vi "DELETE_clear_error_bulk.vi"(8 "API Key":string="cheia04042025tema2restfulapi", 11 "url":string="http://localhost:5000/ecu?param=clear_error_memory") -> (0 "delete_error_":string, 1 "DELETE_clear_specific_error_header":string)   [LabVIEW 2024]
uses:
  <vilib>/httpClient/LabVIEWHTTPClient.lvlib
panel:
  out "error out delete error memory":errorcluster
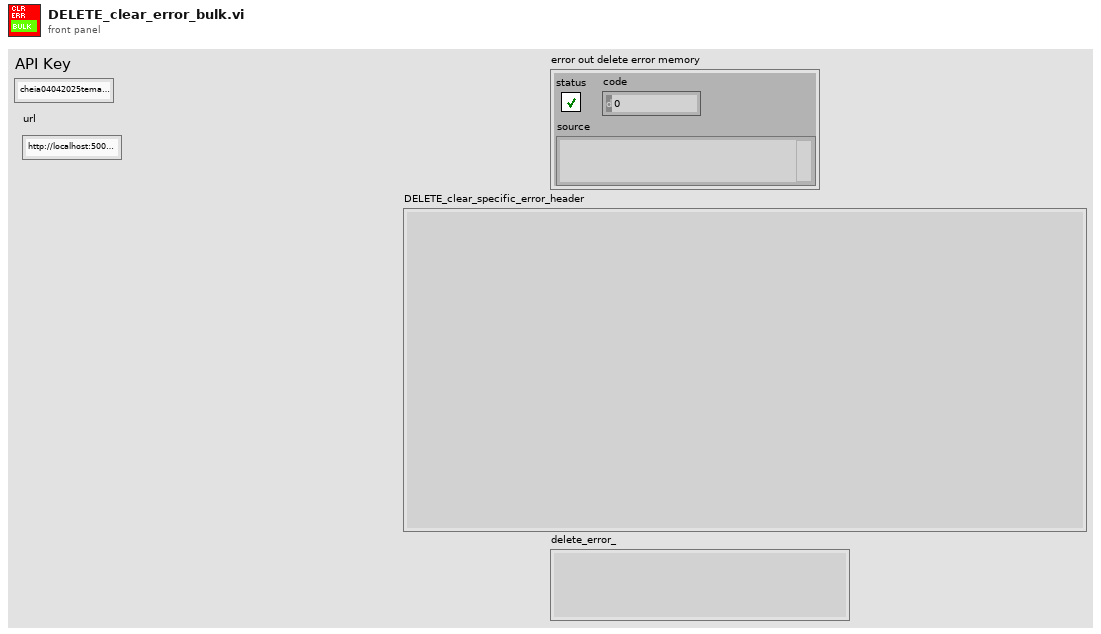
[diagram p1: front panel]
types:
  T1 = typedef "LabVIEWHTTPClient.lvlib/ClientHandle.ctl" = refnum<k1>
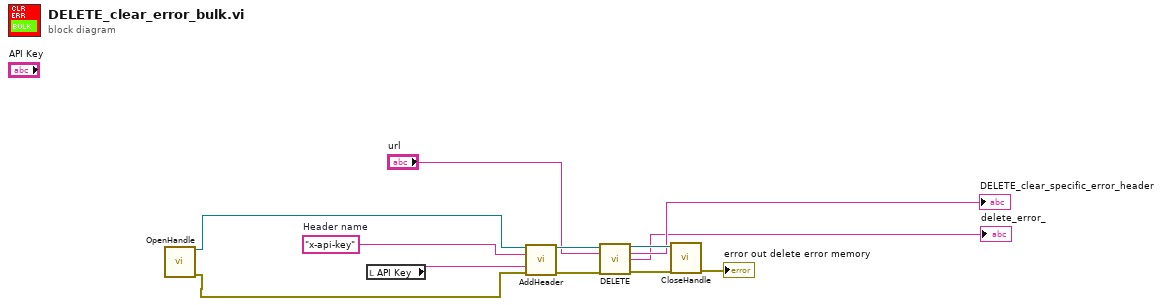
[diagram p0: block diagram]
diagram:
  w4 = "x-api-key"  # Header name
  n1 = call <vilib>:"OpenHandle.vi"() -> ("client handle out"=w6:T1, "error out"=w7:errorcluster)  [unwired: 14 in]
  n2 = local read "API Key"() -> (w3:string)
  n3 = call <vilib>:"AddHeader.vi"("client handle"=w6, "header"=w4, "value"=w3, "error in (no error)"=w7) -> ("client handle out"=w9:T1, "error out"=w8:errorcluster)  [unwired: 10 in]
  n4 = call <vilib>:"DELETE.vi"("client handle"=w9, "url"="url", "error in (no error)"=w8) -> ("client handle out"=w11:T1, "headers"=→"DELETE_clear_specific_error_header":string, "body"=→"delete_error_":string, "error out"=w10:errorcluster)  [unwired: 9 in]
  n5 = call <vilib>:"CloseHandle.vi"("client handle"=w11, "error in (no error)"=w10) -> ("error out"=→"error out delete error memory":errorcluster)  [unwired: 13 in]
